vi "Update Alias in Logger Table.vi"(9 "Device Name":string, 10 "Value":string, 11 "Var Name":string) -> ()   [LabVIEW 2013]
panel:
  in  "Channel_group":string
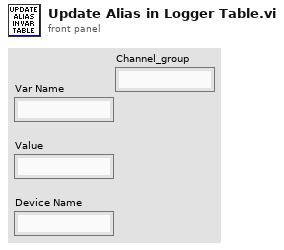
[diagram p1: front panel]
types:
  T1 = typedef "mysql_authentication.ctl" = cluster{"User":string, "Password":string, "Database":string}
  T2 = cluster{"Port":u16, "IP Address":string, "Authentication":T1}
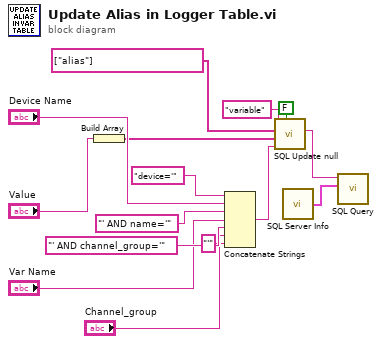
[diagram p0: block diagram]
diagram:
  n1 = Build Array("Value") -> (w7:string[])
  n2 = Concatenate Strings("device='" ("string"), "Device Name", "' AND name='" ("string"), "Var Name", "' AND channel_group='" ("string"), "Channel_group", "'" ("string")) -> (w14:string)
  n3 = call "SQL Update null.vi"("Use Empty String as Ignore? (T)"=FALSE, "Where clause"=w14, "Values"=w7, "Column Names"=string[] ["alias"], "Table"="variable") -> ("Query String"=w8:string)  [unwired: 6 in]
  n4 = call "SQL Server Info.vi"() -> ("SQL Server Info"=w3:T2)
  n5 = call "SQL Query.vi"("SQL Server Info"=w3, "Query"=w8) -> ()  [unwired: 8 in, 2 out]
